vi "SetW12Enabled.vi"(8 "error in (no error)":errorcluster, 10 "w12 enabled":bool, 11 "FpgaRef5761 In":refnum<class "FpgaRef5761.lvclass">) -> (0 "error out":errorcluster, 3 "FpgaRef5761 Out":refnum<class "FpgaRef5761.lvclass">)   [LabVIEW 2018, in "FpgaRef5761.lvclass"]
uses:
  FpgaRef5761.lvclass
  FpgaRef5761.lvclass/FpgaRef5761.ctl
  <vilib>/Utility/error.llb/Error Cluster From Error Code.vi
  <vilib>/rvi/errors/niLvFpgaAdjustHostInterfaceError.vi
  <vilib>/rvi/interface/nirviReadWriteControl/nirviReadWriteControl.xnode
  5761 FPGA ref.ctl
  NiFpgaLv.dll
  <vilib>/rvi/interface/Simulation/niFpgaSimulationCallBeginRW.vi
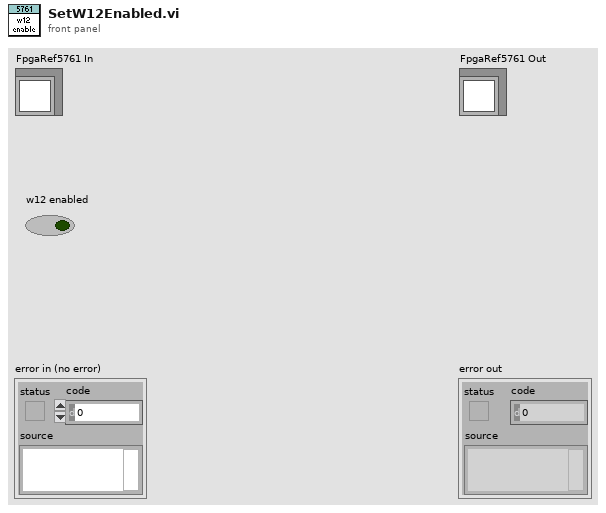
[diagram p1: front panel]
types:
  T1 = typedef "5761 FPGA ref.ctl" = refnum<k20>
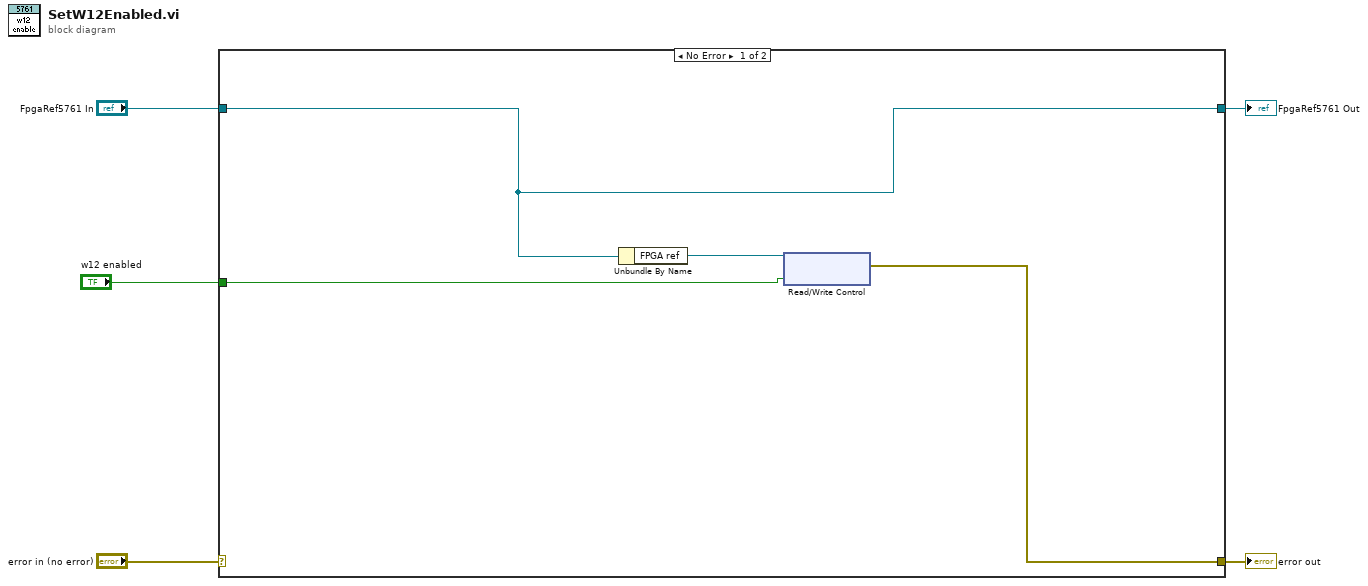
[diagram p0: block diagram]
diagram:
  n1 = case shown="No Error" "error in (no error)" {
    selector: "error in (no error)" -> [_ w11]
    tunnel: [w6 w11] -> w4
    tunnel: [w8 w10] -> w2
    tunnel: "FpgaRef5761 In" -> [w8 w10]
    tunnel: "w12 enabled" -> [w7 _]
    frame No Error {
      n2 = Unbundle By Name(w8) -> ("FPGA ref"=w9:T1)
      n3 = xnode "Read/Write Control"("FPGA VI Reference In"=w9, "W12 enabled"=w7) -> ("error out"=w6:errorcluster)  [unwired: 1 in, 1 out]
    }
    frame Error {
    }
  }
  "error out" <- w4
  "FpgaRef5761 Out" <- w2
